vi "Init Data.vi"(10 "Connector Type":T1) -> (2 "Data":T2 {"Input sources" items=["--unused--", "Probe Mic Right", "Probe Mic Left", "Cal Mic", "ABR", "CAP Right", "CAP Left", "Startle piezo", "Temperature", "Heart rate", "Accelerometer", "Startle piezo 2"]; "Output sources" items=["--unused--", "Right primary", "Right secondary", "Left primary", "Left secondary", "Shocks", "Startle", "Background", "Shaker", "Blue laser"]})   [LabVIEW 2020, in "PXISlot.xctl"]
uses:
  PXISlot.xctl
  Data.ctl
  Output sources.ctl
  Input sources.ctl
  Connector Type.ctl
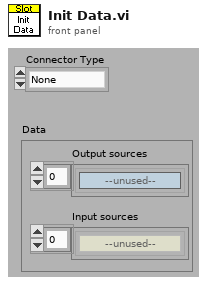
[diagram p1: front panel]
types:
  T1 = typedef "Connector Type.ctl" = enum16{"None", "PXI-4461", "BNC-2110", "BNC-2090", "PXIe-4463", "PXIe-4464"}
  T2 = typedef "PXISlot.xctl/Data.ctl" = cluster{"Output sources":T3[], "Input sources":T4[]}
  T3 = typedef "Output sources.ctl" = u16
  T4 = typedef "Input sources.ctl" = u16
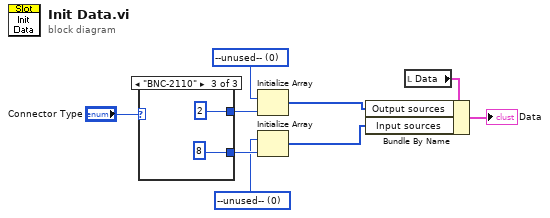
[diagram p0: block diagram]
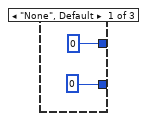
[diagram p2: hidden frame]
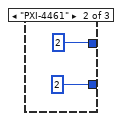
[diagram p3: hidden frame]
diagram:
  w2 = T4 0 items=["--unused--", "Probe Mic Right", "Probe Mic Left", "Cal Mic", "ABR", "CAP Right", "CAP Left", "Startle piezo", "Temperature", "Heart rate"] ("Ring")
  w3 = T3 0 items=["--unused--", "Right primary", "Right secondary", "Left primary", "Left secondary", "Shocks", "Startle", "Background"] ("Ring")
  n1 = case shown="\"BNC-2110\"" "Connector Type" {
    tunnel: [0 2 2] -> w8
    tunnel: [0 2 8] -> w7
    frame "None", Default {
    }
    frame "PXI-4461" {
    }
    frame "BNC-2110" {
    }
  }
  n2 = Initialize Array(w3, w8) -> (w5:T3[])
  n3 = Initialize Array(w2, w7) -> (w4:T4[])
  n4 = local read "Data"() -> (w6:T2)
  n5 = Bundle By Name(cluster=w6, "Output sources"=w5, "Input sources"=w4) -> (→"Data":T2)
